vi "Msg To.vi"(10 "String Indicator":string) -> (3 "String Indicator Msg Strategy out":refnum<class "String Indicator Msg Strategy.lvclass">)   [LabVIEW 2021, in "String Indicator.lvlib"]
uses:
  String Indicator.lvlib
  String Indicator Msg Strategy/String Indicator Msg Strategy.lvclass
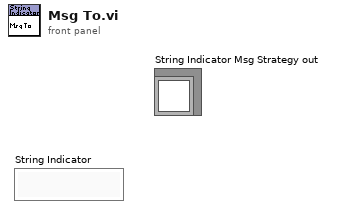
[diagram p1: front panel]
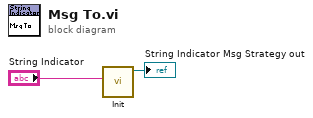
[diagram p0: block diagram]
diagram:
  n1 = call "Init.vi"("String Indicator"="String Indicator") -> ("String Indicator Msg Strategy out"=→"String Indicator Msg Strategy out":refnum<class "String Indicator Msg Strategy.lvclass">)  [unwired: 10 in]
